vi "FaceTrackingFromCamera.vi"   [LabVIEW 2019]
doc: "This example demonstrates the Traditional MeanShift algorithm to track an object in the image."
panel:
  # "Overview: Demonstrate the Traditional MeanShift algorithm to track an object in the image.\nRequirements: LabVIEW Full Development System and Vision Development Module.\nInstructions: Run the VI."
types:
  T1 = cluster{"Number of Histogram Bins":i32, "Blending Parameter (%)":dbl, "Maximum Iterations":i32}
  T2 = typedef "IMAQ Object Tracking Session.ctl" = refnum<k20>
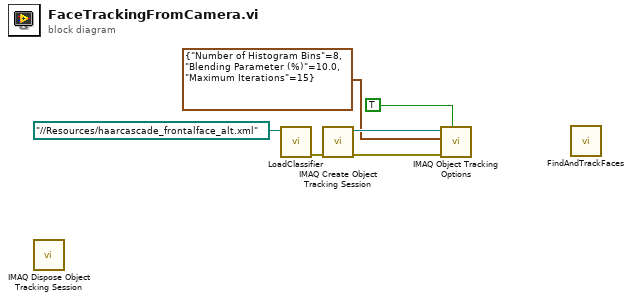
[diagram p0: block diagram]
diagram:
  n1 = call "IMAQ Dispose Object Tracking Session"() -> ()  [unwired: 2 in, 10 out]
  n2 = call "LoadClassifier.vi"("faceCascadePath"=path "../../Resources/haarcascade_frontalface_alt.xml" ("Face Cascade Path")) -> ("error out"=w1:errorcluster)  [unwired: 10 in]
  n3 = call "IMAQ Create Object Tracking Session"("error in (no error)"=w1) -> ("error out"=w4:errorcluster, "Object Tracking Session"=w6:T2)  [unwired: 9 out]
  n4 = call-poly "IMAQ Object Tracking Options"("Get/Set (Get)"=TRUE, "error in (no error)"=w4, "Mean Shift Options in"=T1 {"Number of Histogram Bins"=8, "Blending Parameter (%)"=10.0, "Maximum Iterations"=15}, "Object Tracking Session In"=w6) -> ()  [unwired: 5 in, 3 out]
  n5 = call "FindAndTrackFaces.vi"() -> ()  [unwired: 8 in, 4 out]
